vi "execution class name.vi"(8 "error in":errorcluster, 11 "configuration in":refnum<class "fixed channel configuration.lvclass">) -> (0 "error out":errorcluster, 2 "execution class":string, 3 "configuration out":refnum<class "fixed channel configuration.lvclass">)   [LabVIEW 2013, in "fixed channel configuration.lvclass"]
uses:
  fixed channel configuration.lvclass
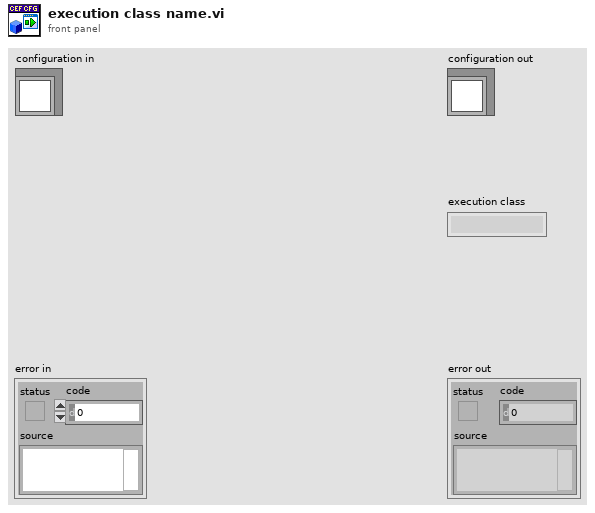
[diagram p1: front panel]
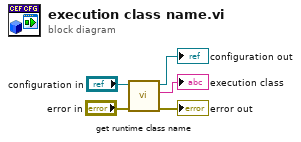
[diagram p0: block diagram]
diagram:
  n1 = call-dynamic "get runtime class name.vi"("error in"="error in", "fixed module parent implementation configuration in"="configuration in") -> ("error out"=→"error out":errorcluster, "class name"=→"execution class":string, "fixed module parent implementation configuration out"=→"configuration out":refnum<class "fixed channel configuration.lvclass">)  [unwired: 7 in]
